vi "dateTempClusterProvider.vi"(3 "Time Stamp":timestamp format="%<%X\n%x>T") -> (1 "Cluster":cluster{"Time Stamp":timestamp, "Numeric":i32} {"Time Stamp" format="%<%X\n%x>T"})   [LabVIEW 2017]
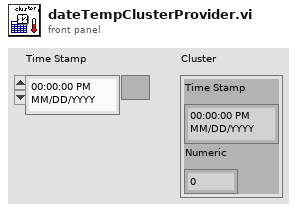
[diagram p1: front panel]
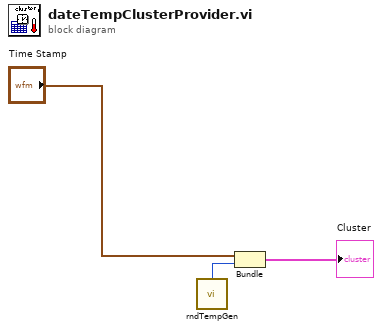
[diagram p0: block diagram]
diagram:
  n1 = call "rndTempGen.vi"() -> ("Numeric"=w1:i32)  [unwired: 11 in]
  n2 = Bundle("Time Stamp"="Time Stamp", "Numeric"=w1) -> (→"Cluster":cluster{"Time Stamp":timestamp, "Numeric":i32})  [unwired: 1 in]
